vi "Write Forward Drive Status.vi"(8 "error in (no error)":errorcluster, 10 "Forward Drive Status":T1 {"Right Drive Power" min=-1.0 max=1.0 scale=-1.0..1.0; "Left Drive Power" min=-1.0 max=1.0 scale=-1.0..1.0}, 11 "Forward Drive Cmd in":refnum<class "Forward Drive Cmd.lvclass">) -> (0 "error out":errorcluster, 3 "Forward Drive Cmd out":refnum<class "Forward Drive Cmd.lvclass">)   [LabVIEW 2014, in "Forward Drive.lvlib" / "Forward Drive Cmd.lvclass"]
uses:
  Forward Drive Cmd.lvclass
  Virtual Robot/Virtual Forward Drive/Virtual Forward Drive Class/Forward Drive State.ctl
  Forward Drive Cmd.lvclass/Forward Drive Cmd.ctl
  Forward Drive Class/Forward Drive.lvclass
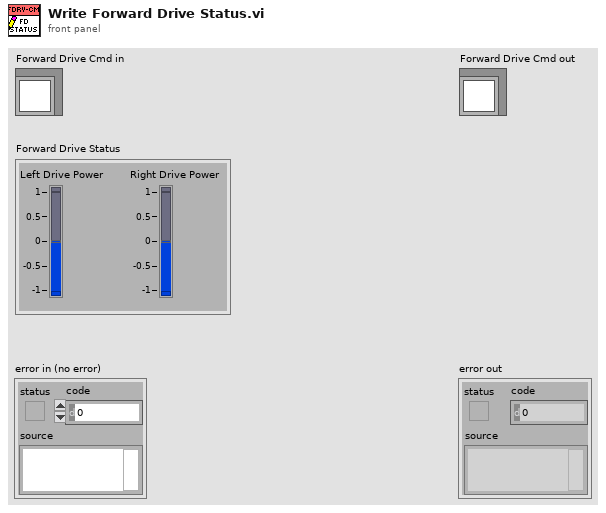
[diagram p1: front panel]
types:
  T1 = typedef "Forward Drive.lvlib/Forward Drive.lvclass/Forward Drive State.ctl" = cluster{"Left Drive Power":dbl, "Right Drive Power ":dbl}
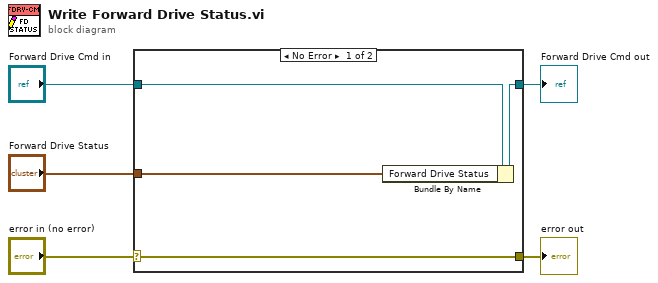
[diagram p0: block diagram]
diagram:
  n1 = case shown="No Error" "error in (no error)" {
    selector: "error in (no error)" -> [w9 w10]
    tunnel: [w9 w10] -> w4
    tunnel: [w7 w11] -> w2
    tunnel: "Forward Drive Cmd in" -> [w8 w11]
    tunnel: "Forward Drive Status" -> [w6 _]
    frame No Error {
      n2 = Bundle By Name(cluster=w8, "Forward Drive Status"=w6) -> (w7:refnum<class "Forward Drive Cmd.lvclass">)
    }
    frame Error {
    }
  }
  "error out" <- w4
  "Forward Drive Cmd out" <- w2
